vi "q5 event structure.vi"() -> ()   [LabVIEW 2018]
panel:
  in  "stop":bool
  in  "DIV":bool
  in  "MUL":bool
  in  "SUB":bool
  in  "ADD":bool
  out "RESULT":dbl
  in  "B":dbl
  in  "A":dbl
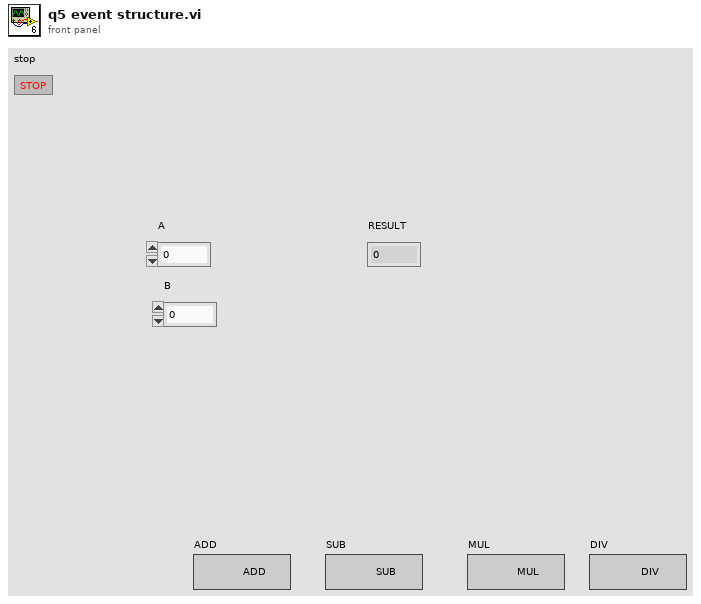
[diagram p1: front panel]
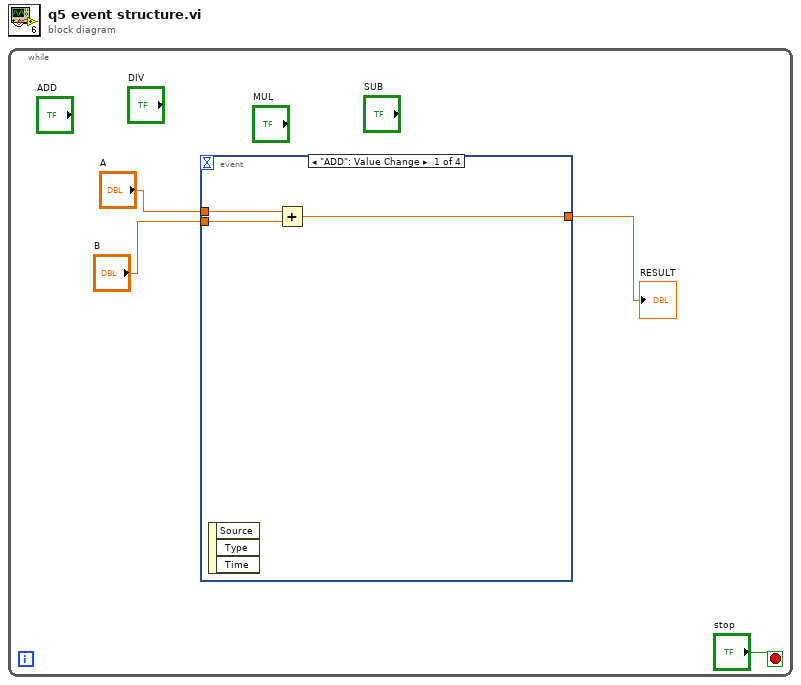
[diagram p0: block diagram]
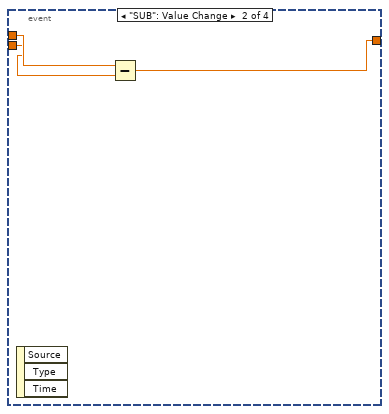
[diagram p2: hidden frame]
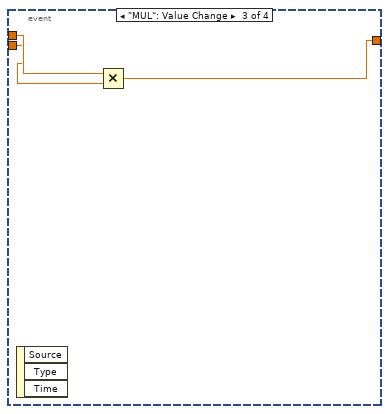
[diagram p3: hidden frame]
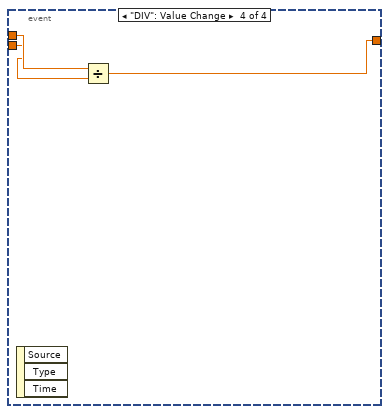
[diagram p4: hidden frame]
diagram:
  n1 = while {
    stop <- "stop" stop-if-true
    n2 = event shown="[0] \"ADD\": Value Change" {
      selector: _ -> [_ _ _ _]
      dyn-events: _ -> [_ _ _ _]
      timeout: _ -> [_ _ _ _]
      tunnel: "A" -> [w7 w10 w13 w16]
      tunnel: "B" -> [w6 w9 w12 w15]
      tunnel: [w5 w8 w11 w14] -> w2
      event "ADD": Value Change {
        n3 = event-data() -> ()  [unwired: 1 in, 3 out]
        n4 = Add(x=w7, y=w6) -> (x+y=w5:dbl)
      }
      event "SUB": Value Change {
        n5 = event-data() -> ()  [unwired: 1 in, 3 out]
        n6 = Subtract(x=w10, y=w9) -> (x-y=w8:dbl)
      }
      event "MUL": Value Change {
        n7 = event-data() -> ()  [unwired: 1 in, 3 out]
        n8 = Multiply(x=w13, y=w12) -> (x*y=w11:dbl)
      }
      event "DIV": Value Change {
        n9 = event-data() -> ()  [unwired: 1 in, 3 out]
        n10 = Divide(x=w16, y=w15) -> (x/y=w14:dbl)
      }
    }
    "RESULT" <- w2
  }
